vi "Get_Button_Position.vi"(0 "Position":T1, 5 "FP_Bounds":T2) -> (4 "Left":i32, 6 "Top":i32)   [LabVIEW 2021]
doc: "Used to get the position of the button."
uses:
  <vilib>/Utility/miscctls.llb/LVRectTypeDef.ctl
  <vilib>/Utility/miscctls.llb/LVPositionTypeDef.ctl
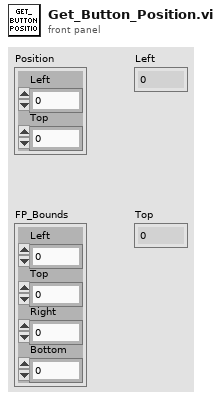
[diagram p1: front panel]
types:
  T1 = typedef "LVPositionTypeDef.ctl" = cluster{"Left":i32, "Top":i32}
  T2 = typedef "LVRectTypeDef.ctl" = cluster{"Left":i16, "Top":i16, "Right":i16, "Bottom":i16}
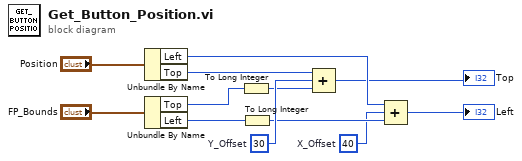
[diagram p0: block diagram]
diagram:
  w12 = 30  # Y_Offset
  w2 = 40  # X_Offset
  n1 = Unbundle By Name("Position") -> ("Left"=w5:i32, "Top"=w6:i32)
  n2 = Unbundle By Name("FP_Bounds") -> ("Top"=w7:i16, "Left"=w9:i16)
  n3 = To Long Integer(number=w7) -> (32bit integer=w8:i32)
  n4 = To Long Integer(number=w9) -> (32bit integer=w10:i32)
  n5 = Compound Arithmetic op=ADD(w6, w12, w8) -> (→"Top":i32)
  n6 = Compound Arithmetic op=ADD(w5, w2, w10) -> (→"Left":i32)
